vi "Spread Histogram.vi"(0 "Array in":dbl[][](array[numeric]), 5 "Min":dbl, 7 "Max":dbl) -> (4 "Array out":dbl[][](array[numeric]))   [LabVIEW 2014]
doc: "Spreads the values of the input Array in to fit the borders Min and Max."
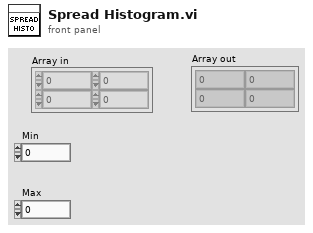
[diagram p1: front panel]
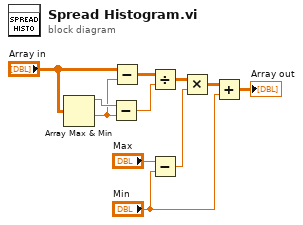
[diagram p0: block diagram]
diagram:
  n1 = Array Max & Min(array="Array in") -> (max value=w8:dbl, min value=w1:dbl)  [unwired: 2 out]
  n2 = Subtract(x=w8, y=w1) -> (x-y=w10:dbl)
  n3 = Subtract(x="Array in", y=w1) -> (x-y=w9:dbl[][])
  n4 = Divide(x=w9, y=w10) -> (x/y=w11:dbl[][])
  n5 = Subtract(x="Max", y="Min") -> (x-y=w6:dbl)
  n6 = Multiply(x=w11, y=w6) -> (x*y=w5:dbl[][])
  n7 = Add(x=w5, y="Min") -> (x+y=→"Array out":dbl[][])
